vi "Kafka_GetData.vi"(8 "error in (no error)":errorcluster, 11 "Consumer Handle":string="localhost:9092") -> (0 "error out":errorcluster, 2 "Events":T1[](array[typedef]), 3 "Consumer Handle":string)   [LabVIEW 2019, in "LVKafka.lvlib"]
uses:
  LVKafka.lvlib
  KafkaConsumerEvent.ctl
  KafkaLVLib.dll
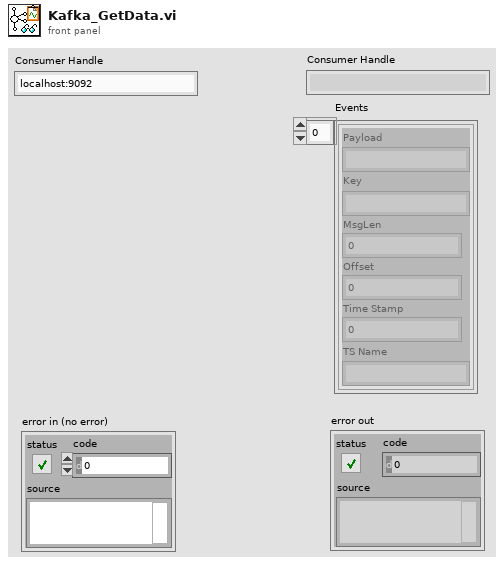
[diagram p1: front panel]
types:
  T1 = typedef "LVKafka.lvlib/KafkaConsumerEvent.ctl" = cluster{"Payload":string, "Key":string, "MsgLen":u64, "Offset":i64, "Time Stamp":i64, "TS Name":string}
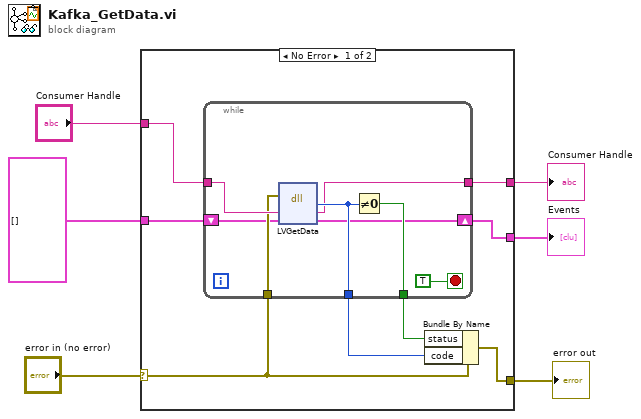
[diagram p0: block diagram]
diagram:
  n1 = case shown="No Error" "error in (no error)" {
    selector: "error in (no error)" -> [w10 w25]
    tunnel: "Consumer Handle" -> [w11 w23]
    tunnel: [w12 w25] -> w4
    tunnel: [w9 w23] -> w3
    tunnel: [w8 w24] -> w2
    tunnel: T1[] [] ("Events 2") -> [w7 w24]
    frame No Error {
      n2 = while {
        tunnel: [w22] -> w14
        tunnel: [w21] -> w13
        tunnel: w10 -> [w19]
        tunnel: w11 -> [w20]
        tunnel: [w18] -> w9
        shift-right: [w16] -> w8
        shift-left: w7 -> [w15]
        stop <- TRUE stop-if-true
        n3 = dll-call lib="KafkaLVLib.*" fn="LVGetData"(error in=w19, "consumerhandle"=w20, "events"=w15) -> ("error"=w21:i32, "consumerhandle"=w18:string, "events"=w16:T1[])  [unwired: 2 in, 2 out]
        n4 = Not Equal To 0?(x=w21) -> (x != 0?=w22:bool)
      }
      n5 = Bundle By Name(cluster=w10, "status"=w14, "code"=w13) -> (w12:errorcluster)
    }
    frame Error {
    }
  }
  "error out" <- w4
  "Consumer Handle" <- w3
  "Events" <- w2
